vi "HW_Acquisition_Start.vi"(2 "Error In":errorcluster, 3 "VISA resource name in":refnum<visa-resource-name>) -> (0 "Error Out":errorcluster, 1 "VISA resource name out":refnum<visa-resource-name>)   [LabVIEW 2018]
uses:
  <vilib>/Instr/_visa.llb/VISA Flush IO Buffer Mask.ctl
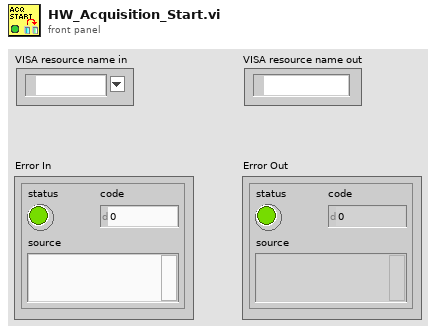
[diagram p1: front panel]
types:
  T1 = typedef "VISA Flush IO Buffer Mask.ctl" = u16
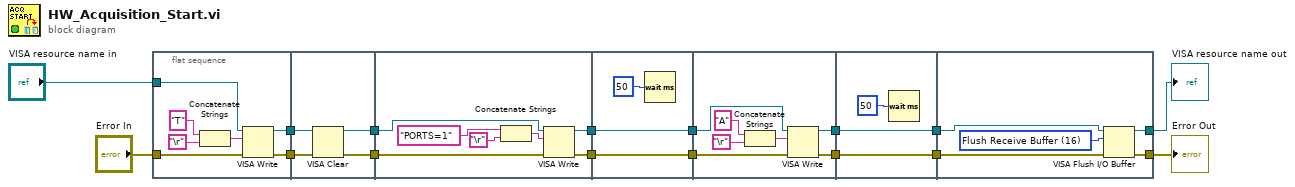
[diagram p0: block diagram]
diagram:
  n1 = flat-sequence {
    tunnel: "VISA resource name in" -> [w22]
    tunnel: [w23] -> w15
    tunnel: [w21] -> w16
    tunnel: "Error In" -> [w17]
    tunnel: [w27] -> w14
    tunnel: [w26] -> w13
    tunnel: w16 -> [w25]
    tunnel: w15 -> [w24]
    tunnel: w14 -> [w32]
    tunnel: [w31] -> w12
    tunnel: w13 -> [w30]
    tunnel: [w29] -> w11
    tunnel: [w37] -> w10
    tunnel: [w36] -> w9
    tunnel: w12 -> [w37]
    tunnel: w11 -> [w36]
    tunnel: [w39] -> w7
    tunnel: [w38] -> w8
    tunnel: w10 -> [w41]
    tunnel: w9 -> [w40]
    tunnel: [w47] -> w5
    tunnel: [w46] -> w6
    tunnel: w8 -> [w46]
    tunnel: w7 -> [w47]
    tunnel: [w52] -> w4
    tunnel: [w51] -> w1
    tunnel: w6 -> [w48]
    tunnel: w5 -> [w49]
    frame #0 {
      n2 = Concatenate Strings("T" ("write buffer"), "\r") -> (w18:string)
      n3 = VISA Write(VISA resource name=w22, write buffer=w18, error in (no error)=w17) -> (VISA resource name out=w23:refnum<visa-resource-name>, error out=w21:errorcluster)  [unwired: 1 out]
    }
    frame #1 {
      n4 = VISA Clear(VISA resource name=w24, error in (no error)=w25) -> (VISA resource name out=w27:refnum<visa-resource-name>, error out=w26:errorcluster)
    }
    frame #2 {
      n5 = Concatenate Strings("PORTS=1" ("write buffer"), "\r") -> (w33:string)
      n6 = VISA Write(VISA resource name=w32, write buffer=w33, error in (no error)=w30) -> (VISA resource name out=w31:refnum<visa-resource-name>, error out=w29:errorcluster)  [unwired: 1 out]
    }
    frame #3 {
      n7 = Wait (ms)(milliseconds to wait=u32 50) -> ()  [unwired: 1 out]
    }
    frame #4 {
      n8 = Concatenate Strings("A" ("write buffer"), "\r") -> (w42:string)
      n9 = VISA Write(VISA resource name=w41, write buffer=w42, error in (no error)=w40) -> (VISA resource name out=w38:refnum<visa-resource-name>, error out=w39:errorcluster)  [unwired: 1 out]
    }
    frame #5 {
      n10 = Wait (ms)(milliseconds to wait=u32 50) -> ()  [unwired: 1 out]
    }
    frame #6 {
      w50 = T1 16 items=["Flush Receive Buffer"=16, "Write Transmit Buffer to Device"=32, "Flush Receive Buffer (No I/O)"=64, "Flush Transmit Buffer"=128] ("Mask")
      n11 = VISA Flush I/O Buffer(VISA resource name=w48, mask (16)=w50, error in (no error)=w49) -> (VISA resource name out=w52:refnum<visa-resource-name>, error out=w51:errorcluster)
    }
  }
  "VISA resource name out" <- w4
  "Error Out" <- w1
